vi "rx test.vi"() -> ()   [LabVIEW 2011]
panel:
  out "Correct Frames":i32
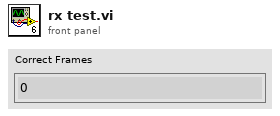
[diagram p1: front panel]
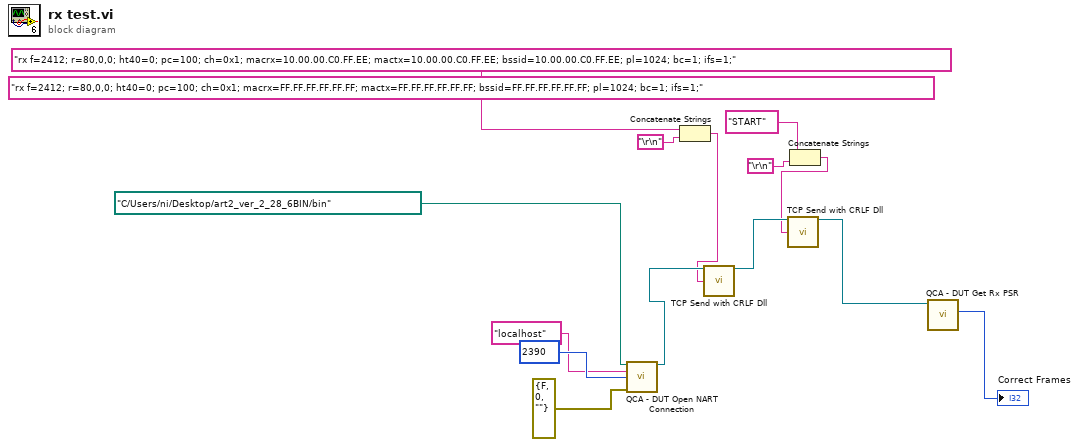
[diagram p0: block diagram]
diagram:
  (unwired) "rx f=2412; r=80,0,0; ht40=0; pc=100; ch=0x1; macrx=FF.FF.FF.FF.FF.FF; mactx=FF.FF.FF.FF.FF.FF; bssid=FF.FF.FF.FF.FF.FF; pl=1024; bc=1; ifs=1;" ("Command Sent")
  n1 = call "QCA - DUT Open NART Connection.vi"("NART Directory"=path "C:/Users/ni/Desktop/art2_ver_2_28_6BIN/bin", "IP Address (\"\": localhost)"="localhost" ("IP Address (\"\": localhost)"), "port (2390)"=u32 2390, "error in (no error)"=errorcluster {"status"=FALSE, "code"=0, "source"=""}) -> ("NART TCP Connection"=w9:refnum<k5>)  [unwired: 10 in, 1 out]
  n2 = Concatenate Strings("rx f=2412; r=80,0,0; ht40=0; pc=100; ch=0x1; macrx=10.00.00.C0.FF.EE; mactx=10.00.00.C0.FF.EE; bssid=10.00.00.C0.FF.EE; pl=1024; bc=1; ifs=1;" ("Command Sent"), "\r\n") -> (w7:string)
  n3 = call "TCP Send with CRLF Dll.vi"("CART TCP Connection"=w9, "CommandIn"=w7) -> ("CART TCP Connection Out"=w6:refnum<k5>)  [unwired: 13 in]
  n4 = Concatenate Strings("START" ("string"), "\r\n") -> (w3:string)
  n5 = call "TCP Send with CRLF Dll.vi"("CART TCP Connection"=w6, "CommandIn"=w3) -> ("CART TCP Connection Out"=w5:refnum<k5>)  [unwired: 13 in]
  n6 = call "QCA - DUT Get Rx PSR.vi"("CART TCP Connection In"=w5) -> ("Correct Frames"=→"Correct Frames":i32)  [unwired: 9 in, 1 out]
